vi "write_attributes.vi"(8 "error in (no error)":errorcluster, 10 "attributes":T1, 11 "ExtraTreesRegressor in":refnum<class "ExtraTreesRegressor.lvclass">) -> (0 "error out":errorcluster, 3 "ExtraTreesRegressor out":refnum<class "ExtraTreesRegressor.lvclass">)   [LabVIEW 2020, in "ExtraTreesRegressor.lvclass"]
uses:
  ExtraTreesRegressor.lvclass
  Controls/extra_trees_regressor_attributes.ctl
  ExtraTreesRegressor.lvclass/ExtraTreesRegressor.ctl
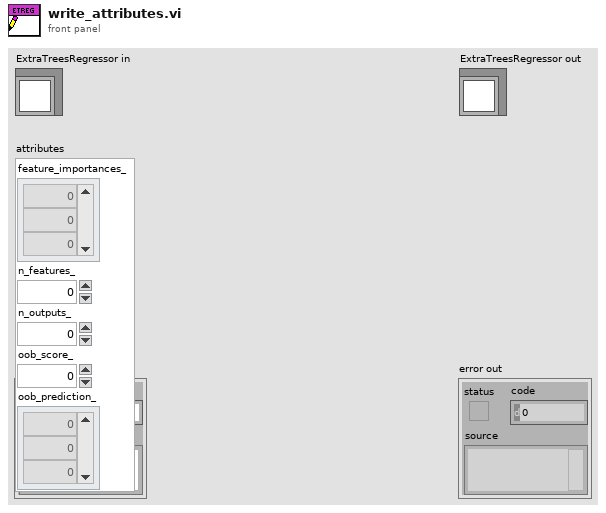
[diagram p1: front panel]
types:
  T1 = typedef "extra_trees_regressor_attributes.ctl" = cluster{"feature_importances_":dbl[], "n_features_":dbl, "n_outputs_":dbl, "oob_score_":dbl, "oob_prediction_":dbl[]}
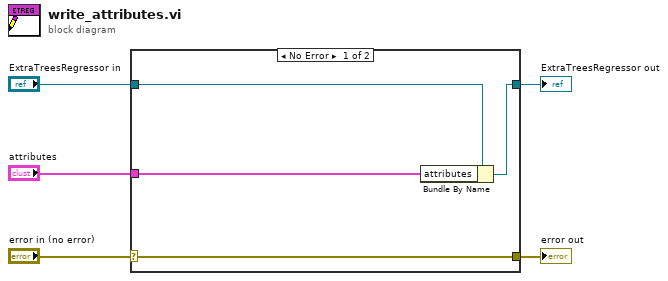
[diagram p0: block diagram]
diagram:
  n1 = case shown="No Error" "error in (no error)" {
    selector: "error in (no error)" -> [w9 w10]
    tunnel: [w9 w10] -> w4
    tunnel: [w7 w11] -> w2
    tunnel: "ExtraTreesRegressor in" -> [w8 w11]
    tunnel: "attributes" -> [w6 _]
    frame No Error {
      n2 = Bundle By Name(cluster=w8, "attributes"=w6) -> (w7:refnum<class "ExtraTreesRegressor.lvclass">)
    }
    frame Error {
    }
  }
  "error out" <- w4
  "ExtraTreesRegressor out" <- w2
